vi "list.get_workbook.vi"(8 "error in (no error)":errorcluster, 10 "index":i32, 11 "List in":refnum<class "List.lvclass">) -> (0 "error out":errorcluster, 2 "Workbook":refnum<class "Workbook.lvclass">, 3 "List out":refnum<class "List.lvclass">)   [LabVIEW 2020, in "List.lvclass"]
uses:
  List.lvclass
  Channel/Channel.lvclass/Channel.ctl
  List.lvclass/List.ctl
  Workbook/Workbook.lvclass
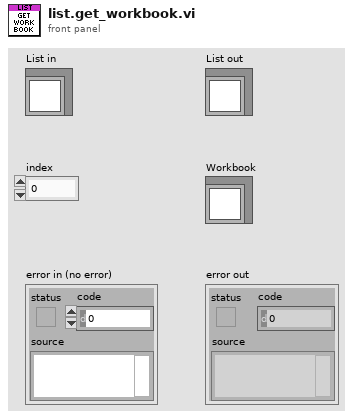
[diagram p1: front panel]
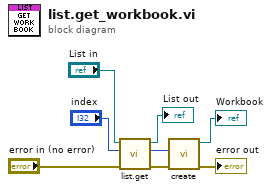
[diagram p0: block diagram]
diagram:
  n1 = call "list.get.vi"("error in"="error in (no error)", "index"="index", "List in"="List in") -> ("error out"=w3:errorcluster, "handle"=w4:i32, "List out"=→"List out":refnum<class "List.lvclass">)  [unwired: 6 in]
  n2 = call "create.vi"("error in (no error)"=w3, "handle"=w4) -> ("error out"=→"error out":errorcluster, "Workbook"=→"Workbook":refnum<class "Workbook.lvclass">)  [unwired: 8 in]
